vi "Layout - Two.vi"(5 "Width (1800)":i32=1800, 7 "Type":T1, 8 "Error in":errorcluster caption="Error in (no error)", 10 "Section 2":string, 11 "Section 1":string) -> (0 "Error out":errorcluster, 3 "Text Output":string)   [LabVIEW 2023, in "Confluence Formatting.lvlib"]
uses:
  Confluence Formatting.lvlib
  Types/Layout - Two Column Type.ctl
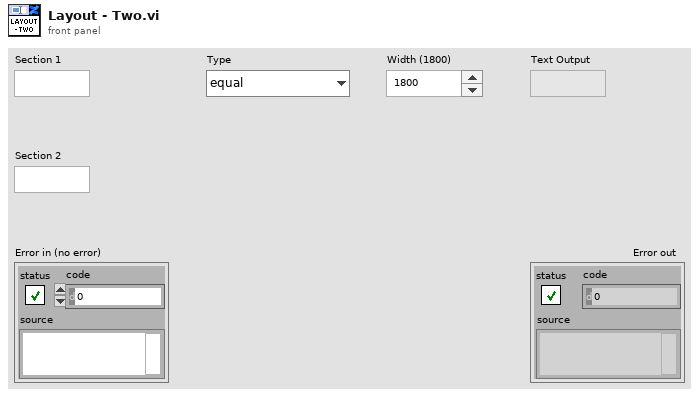
[diagram p1: front panel]
types:
  T1 = typedef "Confluence Formatting.lvlib/Layout - Two Column Type.ctl" = enum16{"equal", "right_sidebar", "left_sidebar"}
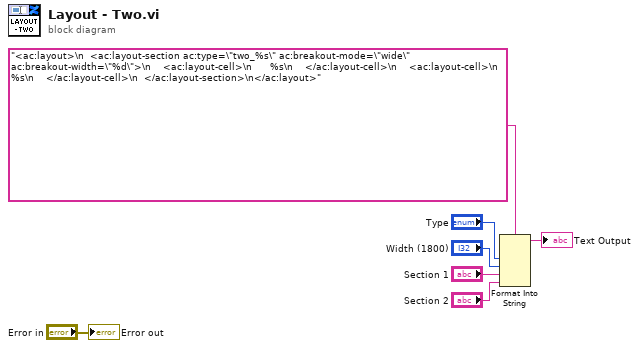
[diagram p0: block diagram]
diagram:
  n1 = Format Into String(format string="<ac:layout>\n  <ac:layout-section ac:type=\"two_%s\" ac:breakout-mode=\"wide\" ac:breakout-width=\"%d\">\n    <ac:layout-cell>\n      %s\n    </ac:layout-cell>\n    <ac:layout-cell>\n      %s\n    </ac:layout-cell>\n  </ac:layout-section>\n</ac:layout>", "Type", "Width (1800)", "Section 1", "Section 2") -> (resulting string=→"Text Output":string)  [unwired: 2 in, 1 out]
  "Error out" <- "Error in"
